vi "Detrend.vi"(8 "Error In":errorcluster, 11 "Smooth Signal Waveform In":waveform(dbl)) -> (0 "Intercept":dbl, 1 "Slope":dbl, 2 "Best Linear Fit":dbl[](array[numeric]), 3 "Detrended Signal Waveform Out":waveform(dbl), 4 "Error Out":errorcluster)   [LabVIEW 2025]
uses:
  <vilib>/Analysis/NI_AALPro.lvlib
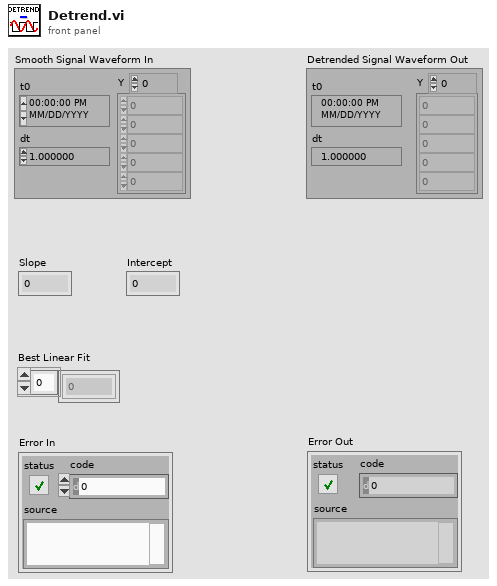
[diagram p1: front panel]
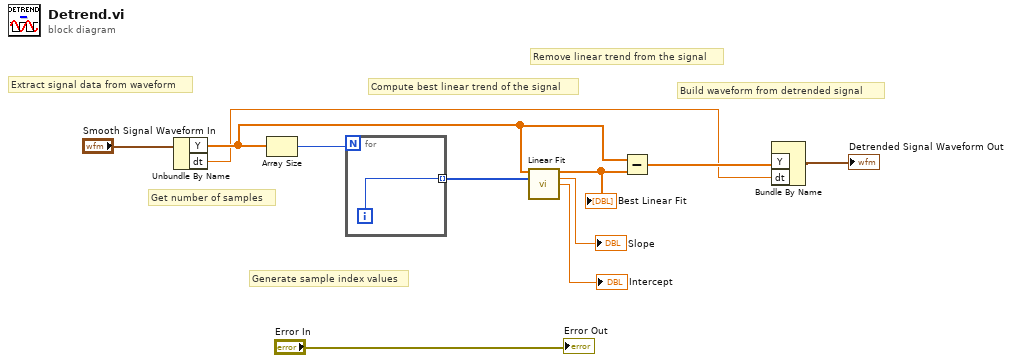
[diagram p0: block diagram]
diagram:
  # "Build waveform from detrended signal"
  # "Remove linear trend from the signal"
  # "Compute best linear trend of the signal"
  # "Generate sample index values"
  # "Get number of samples"
  # "Extract signal data from waveform"
  n1 = Unbundle By Name("Smooth Signal Waveform In") -> ("Y"=w5:dbl[], "dt"=w3:dbl)
  n2 = Array Size(array=w5) -> (size(s)=w10:i32)
  n3 = for {
    N: w10 -> [_]
    tunnel: [w12] -> w11 mode=indexing
    i -> [w12]
  }
  n4 = call <vilib>:"Linear Fit.vi"("Y"=w5, "X"=w11) -> ("Best Linear Fit"=w7:dbl[], "slope"=→"Slope":dbl, "intercept"=→"Intercept":dbl)  [unwired: 9 in, 2 out]
  "Best Linear Fit" <- w7
  n5 = Subtract(x=w5, y=w7) -> (x-y=w4:dbl[])
  n6 = Bundle By Name("Y"=w4, "dt"=w3) -> (→"Detrended Signal Waveform Out":waveform(dbl))  [unwired: 1 in]
  "Error Out" <- "Error In"
